vi "create_instance.vi"(8 "error in (no error)":errorcluster, 11 "relative path":string) -> (0 "error out":errorcluster, 3 "GenericFPGAWrapper out":refnum<class "GenericFPGAWrapper.lvclass">)   [LabVIEW 2010, in "GenericFPGAWrapper.lvclass"]
uses:
  GenericFPGAWrapper.lvclass
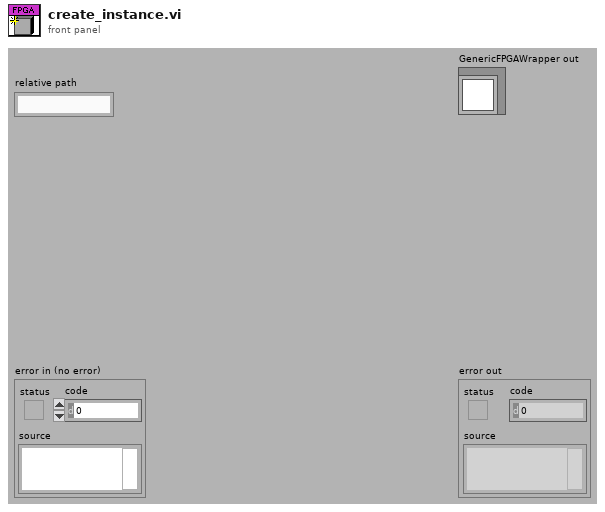
[diagram p1: front panel]
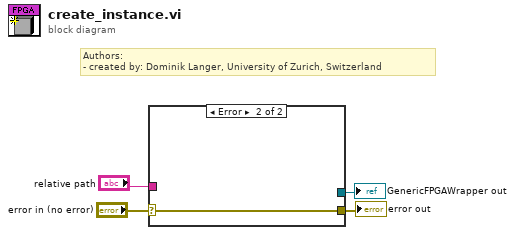
[diagram p0: block diagram]
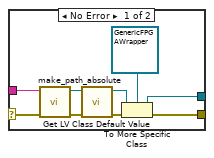
[diagram p2: hidden frame]
diagram:
  # "Authors: \n- created by: Dominik Langer, University of Zurich, Switzerland"
  n1 = case shown="Error" "error in (no error)" {
    selector: "error in (no error)" -> [w11 w14]
    tunnel: [w10 w14] -> w3
    tunnel: [w6 _] -> w2
    tunnel: "relative path" -> [w9 _]
    frame No Error {
      n2 = call "make_path_absolute.vi"("error in (no error)"=w11, "relative path"=w9) -> ("error out"=w12:errorcluster, "absolute path"=w8:path)  [unwired: 8 in]
      n3 = call <vilib>:"Get LV Class Default Value.vi"("error in (no error)"=w12, "class path"=w8) -> ("error out"=w13:errorcluster, "object"=w7:refnum<class>)  [unwired: 8 out]
      n4 = To More Specific Class(target class=refnum<class "GenericFPGAWrapper.lvclass"> refnum ("GenericFPGAWrapper.lvclass"), reference=w7, error in=w13) -> (specific class reference=w6:refnum<class "GenericFPGAWrapper.lvclass">, error out=w10:errorcluster)
    }
    frame Error {
    }
  }
  "error out" <- w3
  "GenericFPGAWrapper out" <- w2
